vi "determine Warnings.vi"() -> ()   [LabVIEW 2014]
panel:
  out "Warning Text":string="Freeze Warning"
  out "Warning?":bool
  in  "Min Temp":dbl
  in  "Max Temp":dbl
  in  "Current Temp":dbl
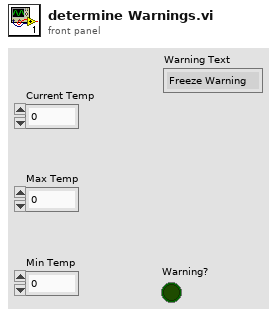
[diagram p1: front panel]
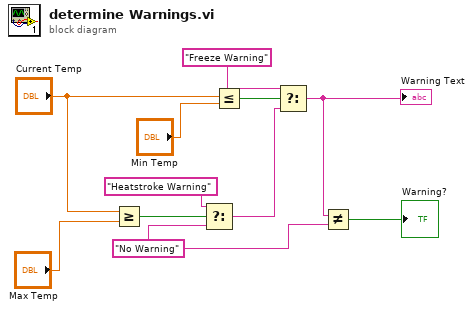
[diagram p0: block diagram]
diagram:
  w3 = "No Warning" ("Warning Text")
  n1 = Greater Or Equal?(x="Current Temp", y="Max Temp") -> (x >= y?=w8:bool)
  n2 = Select(t="Heatstroke Warning" ("Warning Text"), s=w8, f=w3) -> (s? t:f=w4:string)
  n3 = Less Or Equal?(x="Current Temp", y="Min Temp") -> (x <= y?=w6:bool)
  n4 = Select(t="Freeze Warning" ("Warning Text"), s=w6, f=w4) -> (s? t:f=w2:string)
  "Warning Text" <- w2
  n5 = Not Equal?(x=w2, y=w3) -> (x != y?=→"Warning?":bool)
